vi "WriteExample.vi"() -> ()   [LabVIEW 2017]
uses:
  <vilib>/UPVI/lvhdf5/dataspace.llb/H5S_class_t.ctl
  <vilib>/UPVI/lvhdf5/dataspace.llb/H5Screate.vi
  <vilib>/UPVI/lvhdf5/dataspace.llb/H5Screate_simple.vi
  <vilib>/UPVI/lvhdf5/group.llb/OpenCreateGroup (String).vi
  <vilib>/Utility/VariantDataType/GetClusterInfo.vi
  <vilib>/Utility/VariantDataType/GetTypeInfo.vi
  <vilib>/UPVI/lvhdf5/attribute.llb/Write Multiple Attributes.vi
  <vilib>/UPVI/lvhdf5/datatype.llb/LVH5Tcreate_dataset_type (Variant).vi
  <vilib>/UPVI/lvhdf5/dataset.llb/Simple OpenCreateReplace Dataset (Variant).vi
  <vilib>/UPVI/lvhdf5/dataset.llb/H5Dwrite (Variant).vi
  <vilib>/UPVI/lvhdf5/dataset.llb/Append Element(s) to Dataset (Variant).vi
  <vilib>/UPVI/lvhdf5/attribute.llb/LVH5A Operation.ctl
  <vilib>/UPVI/lvhdf5/dataspace.llb/LVH5Screate_matching_space.xnode
  <vilib>/UPVI/lvhdf5/library.llb/HDF5 Ref.ctl
  <vilib>/UPVI/lvhdf5/attribute.llb/LVH5 Write Attributes.xnode
  <vilib>/UPVI/lvhdf5/attribute.llb/Cluster to Attribute Array.xnode
  <vilib>/UPVI/lvhdf5/datatype.llb/LVH5Tcreate_dataset_type.xnode
  <vilib>/UPVI/lvhdf5/dataset.llb/LVH5D Operation.ctl
  <vilib>/UPVI/lvhdf5/dataset.llb/Simple OpenCreateReplace Dataset.xnode
  <vilib>/UPVI/lvhdf5/dataset.llb/H5Dwrite.xnode
  <vilib>/UPVI/lvhdf5/dataset.llb/Append Element(s) to Dataset.xnode
  <vilib>/Utility/VariantDataType/VariantType.lvlib
  <vilib>/UPVI/lvhdf5/dataspace.llb/LVH5Screate_matching_space (Variant).vi
panel:
  in  "path":path
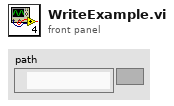
[diagram p1: front panel]
types:
  T1 = typedef "HDF5 Ref.ctl" = refnum<k1>
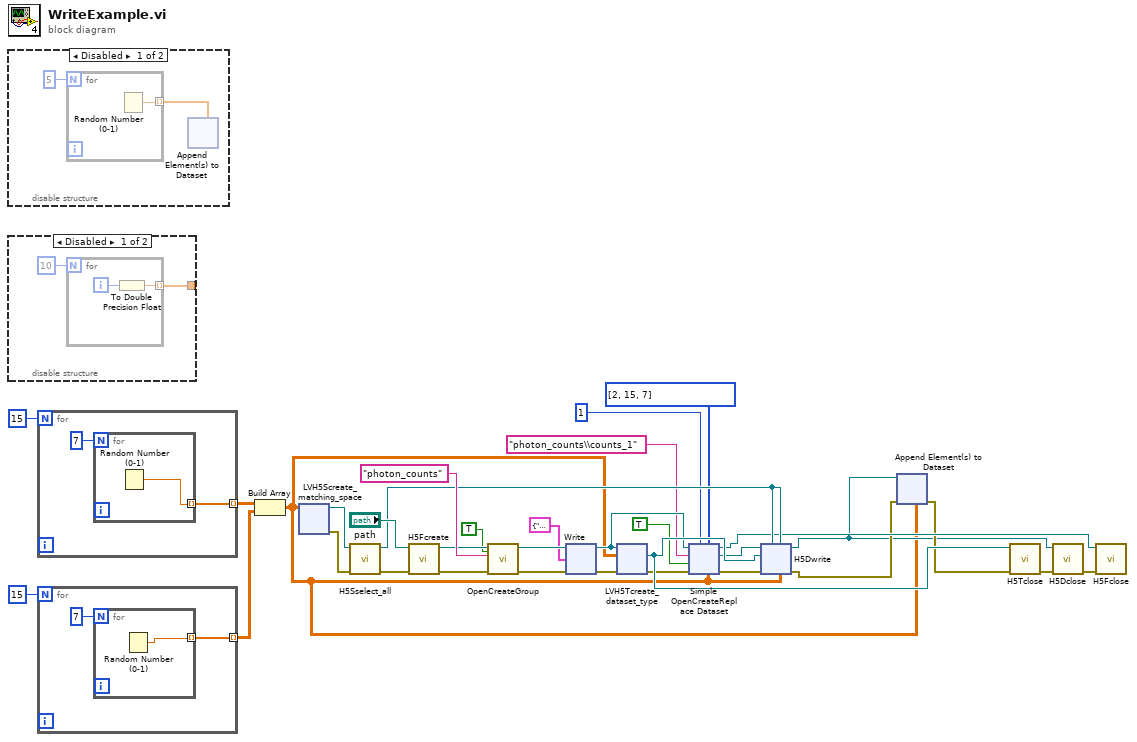
[diagram p0: block diagram]
diagram:
  n1 = disable-structure shown="Disabled" {
    frame Disabled {
      n2 = for {
        N: 5 -> [_]
        tunnel: [w36] -> w34 mode=indexing
        n3 = Random Number (0-1)() -> (number: 0 to 1=w36:dbl)
      }
      n4 = xnode "Append Element(s) to Dataset"("Data Element(s)"=w34) -> ()  [unwired: 3 in, 4 out]
    }
    frame Enabled {
    }
  }
  n5 = disable-structure shown="Disabled" {
    disable-tunnel: [w45 _] -> _
    frame Disabled {
      n6 = for {
        N: 10 -> [_]
        tunnel: [w47] -> w45 mode=indexing
        i -> [w48]
        n7 = To Double Precision Float(number=w48) -> (double precision float=w47:dbl)
      }
    }
    frame Enabled {
    }
  }
  n8 = for {
    N: 15 -> [_]
    tunnel: [w49] -> w15 mode=indexing
    n9 = for {
      N: 7 -> [_]
      tunnel: [w51] -> w49 mode=indexing
      n10 = Random Number (0-1)() -> (number: 0 to 1=w51:dbl)
    }
  }
  n11 = for {
    N: 15 -> [_]
    tunnel: [w52] -> w4 mode=indexing
    n12 = for {
      N: 7 -> [_]
      tunnel: [w54] -> w52 mode=indexing
      n13 = Random Number (0-1)() -> (number: 0 to 1=w54:dbl)
    }
  }
  n14 = Build Array(w15, w4) -> (w3:dbl[][][])
  n15 = xnode "LVH5Screate_matching_space"("Data"=w3) -> ("HDF5 Dataspace Ref"=w25:T1, "error out"=w24:errorcluster)  [unwired: 2 in]
  n16 = call <vilib>:"H5Sselect_all.vi"("error in (no error)"=w24, "HDF5 Space Ref"=w25) -> ("error out"=w22:errorcluster, "HDF5 Ref out"=w18:T1)  [unwired: 6 in]
  n17 = call <vilib>:"H5Fcreate.vi"("error in (no error)"=w22, "path"="path") -> ("error out"=w32:errorcluster, "HDF5 Ref"=w30:T1)  [unwired: 6 in]
  n18 = call-poly <vilib>:"OpenCreateGroup.vi"("Create if not found (F)"=TRUE, "error in (no error)"=w32, "Group"="photon_counts", "HDF5 Ref"=w30) -> ("error out"=w27:errorcluster, "HDF5 Ref out"=w28:T1)  [unwired: 5 in, 1 out]
  n19 = xnode "Write"("HDF5 Ref"=w28, "error in (no error)"=w27, "Value(s)"=cluster{"func":string, "steps":i32} {"func"="statedet", "steps"=0}) -> ("HDF5 Ref out"=w13:T1, "error out"=w23:errorcluster)  [unwired: 2 in]
  n20 = xnode "LVH5Tcreate_dataset_type"("HDF5 Location Ref"=w13, "error in (no error)"=w23, "Data"=w3) -> ("HDF5 Type Ref"=w19:T1, "error out"=w10:errorcluster)  [unwired: 3 in, 3 out]
  n21 = xnode "Simple OpenCreateReplace Dataset"("Chunk size"=i32[] [2, 15, 7], "Compression Level (0-disabled)"=1, "Dataset Path"="photon_counts\\counts_1", "HDF5 Ref"=w13, "Unlimited  dataset (F)"=TRUE, "error in (no error)"=w10, "Datatype and Dataspace"=w3) -> ("HDF5 Dataset Ref out"=w8:T1, "HDF5 Ref out"=w14:T1, "error out"=w9:errorcluster)  [unwired: 1 in]
  n22 = xnode "H5Dwrite"("HDF5 Dataset Ref"=w8, "HDF5 File Space Ref (H5S_ALL)"=w18, "HDF5 Memory Space Ref (H5S_ALL)"=w18, "HDF5 Type Ref (match data)"=w19, "error in (no error)"=w9, "Data"=w3) -> ("HDF5 Ref out"=w5:T1, "error out"=w7:errorcluster)  [unwired: 1 in]
  n23 = xnode "Append Element(s) to Dataset"("HDF5 Dataset Ref"=w5, "error in (no error)"=w7, "Data Element(s)"=w3) -> ("error out"=w6:errorcluster)  [unwired: 1 in, 3 out]
  n24 = call <vilib>:"H5Tclose.vi"("error in (no error)"=w6, "HDF5 Datatype Ref"=w19) -> ("error out"=w20:errorcluster)  [unwired: 7 in]
  n25 = call <vilib>:"H5Dclose.vi"("error in (no error)"=w20, "HDF5 Dataset Ref"=w5) -> ("error out"=w21:errorcluster)  [unwired: 7 in]
  n26 = call <vilib>:"H5Fclose.vi"("error in (no error)"=w21, "HDF5 Ref"=w14) -> ()  [unwired: 7 in, 1 out]
